vi "Open Application Reference.vi"(6 "timeout ms (60000)":i32=60000, 8 "error in (no error)":errorcluster, 9 "port number or service name (3363)":u16=3363, 10 "machine name (\"localhost\")":string="localhost", 11 "App Control API in":refnum<class "AppControlAPI.lvclass">) -> (0 "error out":errorcluster, 3 "App Control API out":refnum<class "AppControlAPI.lvclass">)   [LabVIEW 2018, in "AppControlAPI.lvclass"]
uses:
  AppControlAPI.lvclass
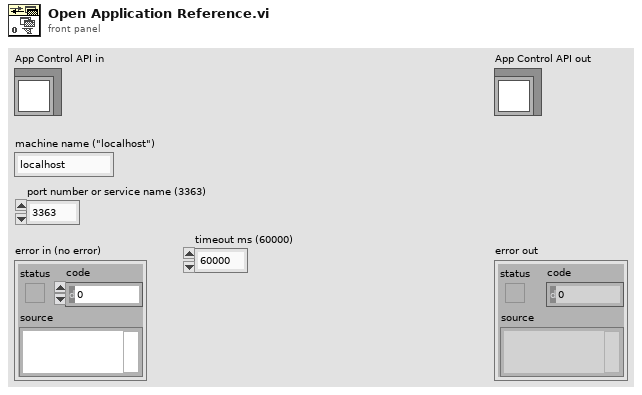
[diagram p1: front panel]
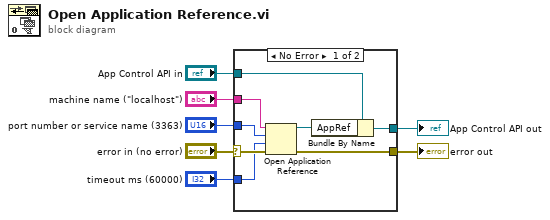
[diagram p0: block diagram]
diagram:
  n1 = case shown="No Error" "error in (no error)" {
    selector: "error in (no error)" -> [w12 w17]
    tunnel: [w9 w17] -> w6
    tunnel: [w11 w16] -> w4
    tunnel: "App Control API in" -> [w15 w16]
    tunnel: "machine name (\"localhost\")" -> [w13 _]
    tunnel: "port number or service name (3363)" -> [w14 _]
    tunnel: "timeout ms (60000)" -> [w8 _]
    frame No Error {
      n2 = Open Application Reference(8:w12, 9:w8, 10:w14, 11:w13) -> (0:w9:errorcluster, 3:w10:refnum<vi>)
      n3 = Bundle By Name(cluster=w15, "AppRef"=w10) -> (w11:refnum<class "AppControlAPI.lvclass">)
    }
    frame Error {
    }
  }
  "error out" <- w6
  "App Control API out" <- w4
